vi "ACC.vi"(0 "System no.":i32=1 min=1 max=4 step=1, 2 "Axes to set":string[](array[string]), 3 "Acceleration values":dbl[](array[numeric]) format="%.6f", 4 "No.of digits":i16=4, 5 "error in":errorcluster, 6 "Without axis ID?":bool) -> (14 "Controller error":bool, 19 "error out":errorcluster)   [LabVIEW 2020]
doc: "Sets closed-loop acceleration and checks for error. If Without axis ID? is TRUE, then Axes to set is ignored and first field of Acceleration values array is used for acceleration command. Number of digits is the number of digits after the decimal point in the acceleration value(s) that will be sent. Controller error is TRUE if selected system reports error code which is not 0.\n\nC-843, C-867, C-877, C-884, C-891, E-861, E-874, Hydra, Pollux, Mercury_GCS: Without axis ID? = FALSE. Acceleration unit is mm/s².\n\nC-413: Without axis ID? = FALSE. Acceleration unit is mm/s².\n\nE-873: Without axis ID? = FALSE. Acceleration unit is mm/s²."
panel:
  # "Sets closed-loop acceleration and checks for error.  If \"Without\naxis ID\" is TRUE, then \"Axes to set\" is ignored and first field of \nAcceleration values\" array is used for acceleration command."
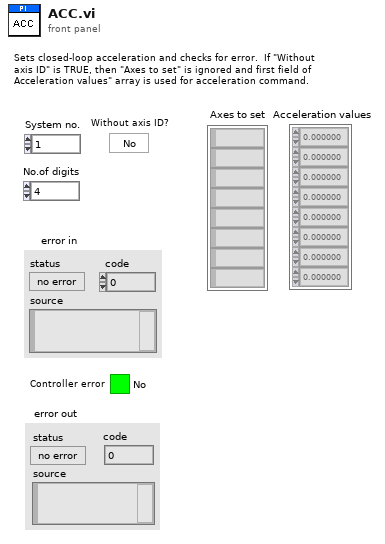
[diagram p1: front panel]
types:
  T1 = enum16{"Disable error check", "Force error check", "Use global settings"}
  T2 = typedef "Syntax.ctl" = enum16{"GCS 1.0", "GCS 2.0", "GCS 3.0"}
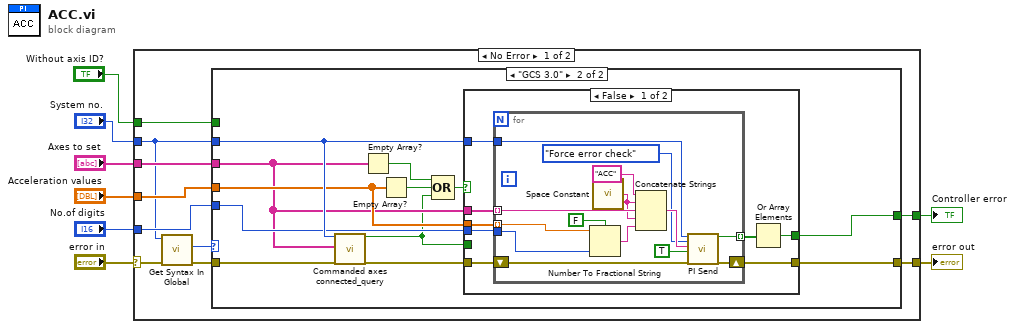
[diagram p0: block diagram]
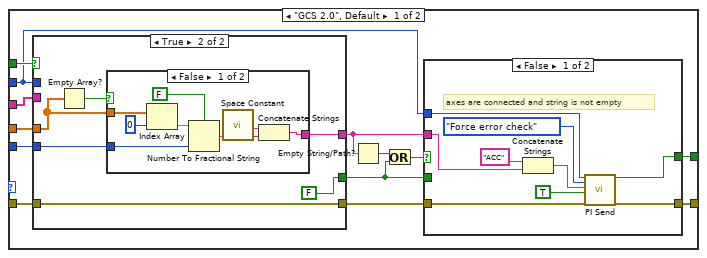
[diagram p2: hidden frame]
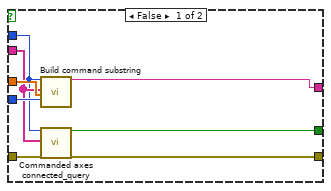
[diagram p3: hidden frame]
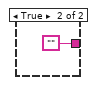
[diagram p4: hidden frame]
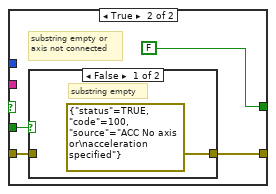
[diagram p5: hidden frame]
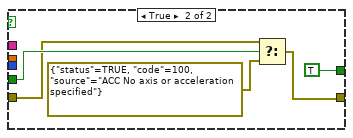
[diagram p7: hidden frame]
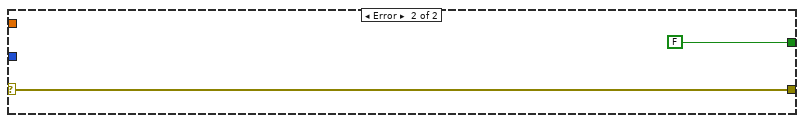
[diagram p8: hidden frame]
diagram:
  n1 = case shown="No Error" "error in" {
    selector: "error in" -> [w11 w109]
    tunnel: [w18 w109] -> w8
    tunnel: "Acceleration values" -> [w17 _]
    tunnel: "No.of digits" -> [w16 _]
    tunnel: "System no." -> [w9 _]
    tunnel: "Axes to set" -> [w15 _]
    tunnel: "Without axis ID?" -> [w14 _]
    tunnel: [w13 FALSE ("Controller error")] -> w1
    frame No Error {
      n2 = call "Get Syntax In Global.vi"("error in"=w11, "System no."=w9) -> ("error out"=w10:errorcluster, "Syntax"=w12:T2)  [unwired: 8 in]
      n3 = case shown="\"GCS 3.0\"" w12 {
        tunnel: [w31 w79] -> w18
        tunnel: w17 -> [w30 w76]
        tunnel: w16 -> [w29 w77]
        tunnel: w15 -> [w27 w75]
        tunnel: w14 -> [w25 _]
        tunnel: w9 -> [w24 w78]
        tunnel: w10 -> [w23 w80]
        tunnel: [w19 w71] -> w13
        frame "GCS 2.0", Default {
          n4 = case shown="True" w25 {
            tunnel: [w39 w43] -> w20
            tunnel: w30 -> [w38 w42]
            tunnel: w29 -> [w37 w40]
            tunnel: w23 -> [w36 w45]
            tunnel: [w35 w45] -> w28
            tunnel: w24 -> [w32 _]
            tunnel: w27 -> [w34 _]
            tunnel: [w33 FALSE] -> w22
            frame False {
              n5 = call "Build command substring.vi"("System no."=w32, "Affected axes"=w34, "Parameters"=w38, "No. of digits"=w37) -> ("Command substring"=w39:string)  [unwired: 3 in, 12 out]
              n6 = call "Commanded axes connected_query.vi"("System no."=w32, "Commanded axes"=w34, "error in"=w36) -> ("Controller error"=w33:bool, "error out"=w35:errorcluster)  [unwired: 1 in, 14 out]
            }
            frame True {
              n7 = Empty Array?(array=w42) -> (empty?=w41:bool)
              n8 = case shown="False" w41 {
                tunnel: [w51 ""] -> w43
                tunnel: w42 -> [w50 _]
                tunnel: w40 -> [w48 _]
                frame False {
                  n9 = Index Array(array=w50, index=0 ("Index")) -> (element=w47:dbl)
                  n10 = Number To Fractional String(use system decimal point (T)=FALSE, number=w47, precision (6)=w48) -> (F-format string=w49:string)  [unwired: 1 out]
                  n11 = call "Space Constant.vi"() -> ("String"=w52:string)
                  n12 = Concatenate Strings(w52, w49) -> (w51:string)
                }
                frame True {
                }
              }
            }
          }
          n13 = Empty String/Path?(string/path=w20) -> (empty?=w21:bool)
          n14 = Or(x=w21, y=w22) -> (x .or. y?=w26:bool)
          n15 = case shown="False" w26 {
            tunnel: w20 -> [w62 _]
            tunnel: [w56 w67] -> w31
            tunnel: w28 -> [w59 w65]
            tunnel: w22 -> [_ w66]
            tunnel: w24 -> [w58 _]
            tunnel: [w55 FALSE ("Controller error")] -> w19
            frame False {
              # "axes are connected and string is not empty"
              n16 = Concatenate Strings("ACC", w62) -> (w60:string)
              n17 = call "PI Send.vi"("System no."=w58, "Error check settings"=T1."Force error check", "String to send"=w60, "Attach termination char.?"=TRUE ("Attach Linefeed?"), "error in"=w59) -> ("Controller error"=w55:bool, "error out"=w56:errorcluster)  [unwired: 1 in, 12 out]
            }
            frame True {
              # "substring empty or\naxis not connected"
              n18 = case shown="False" w66 {
                tunnel: [errorcluster {"status"=TRUE, "code"=100, "source"="ACC No axis or\nacceleration specified"} ("error out") w69] -> w67
                tunnel: w65 -> [_ w69]
                frame False {
                  # "substring empty"
                }
                frame True {
                  # "commanded axis\nnot connected"
                }
              }
            }
          }
        }
        frame "GCS 3.0" {
          n19 = call "Commanded axes connected_query.vi"("System no."=w78, "Commanded axes"=w75, "error in"=w80) -> ("Controller error"=w70:bool, "error out"=w81:errorcluster)  [unwired: 15 out]
          n20 = Empty Array?(array=w75) -> (empty?=w74:bool)
          n21 = Empty Array?(array=w76) -> (empty?=w73:bool)
          n22 = Compound Arithmetic op=OR(w74, w73, w70) -> (w72:bool)
          n23 = case shown="False" w72 {
            tunnel: w81 -> [w89 w106]
            tunnel: [w88 w104] -> w79
            tunnel: w75 -> [w87 _]
            tunnel: w78 -> [w86 _]
            tunnel: w76 -> [w85 _]
            tunnel: w77 -> [w84 _]
            tunnel: [w82 TRUE] -> w71
            tunnel: w70 -> [_ w107]
            frame False {
              n24 = for {
                shift-right: [w103] -> w88
                shift-left: w89 -> [w102]
                tunnel: w87 -> [w98] mode=indexing
                tunnel: w85 -> [w95] mode=indexing
                tunnel: w86 -> [w96]
                tunnel: w84 -> [w93]
                tunnel: [w91] -> w83 mode=indexing
                n25 = Number To Fractional String(use system decimal point (T)=FALSE, number=w95, precision (6)=w93) -> (F-format string=w94:string)  [unwired: 1 in]
                n26 = call "Space Constant.vi"() -> ("String"=w97:string)
                n27 = Concatenate Strings("ACC", w97, w98, w97, w94) -> (w99:string)
                n28 = call "PI Send.vi"("System no."=w96, "Error check settings"=T1."Force error check", "String to send"=w99, "Attach termination char.?"=TRUE ("Attach Linefeed?"), "error in"=w102) -> ("Controller error"=w91:bool, "error out"=w103:errorcluster)  [unwired: 1 in, 12 out]
              }
              n29 = Or Array Elements(Boolean array=w83) -> (logical OR=w82:bool)
            }
            frame True {
              n30 = Select(t=w106, s=w107, f=errorcluster {"status"=TRUE, "code"=100, "source"="ACC No axis or acceleration specified"} ("error out")) -> (s? t:f=w104:errorcluster)
            }
          }
        }
      }
    }
    frame Error {
    }
  }
  "error out" <- w8
  "Controller error" <- w1
